vi "Sort Goal Info.vi"(0 "Distances Info":T2(array[cluster])) -> (1 "Left Goal":T3, 2 "Right Goal":T3)   [LabVIEW 2013]
uses:
  Common Code/Goal Info.ctl
  Vision/Goal Detection/TargetType.ctl
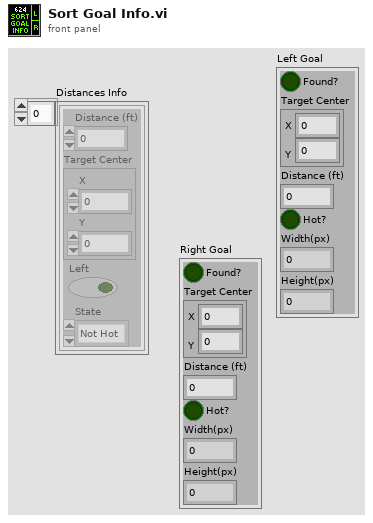
[diagram p1: front panel]
types:
  T1 = typedef "TargetType.ctl" = enum16{"Not Hot", "Hot"}
  T2 = cluster{"Distance (ft)":dbl, "Target Center":cluster{"X":dbl, "Y":dbl}, "Left":bool, "State":T1}[]
  T3 = typedef "Goal Info.ctl" = cluster{"Found?":bool, "Target Center":cluster{"X":dbl, "Y":dbl}, "Distance (ft)":dbl, "Hot?":bool, "Width(px)":dbl, "Height(px)":dbl}
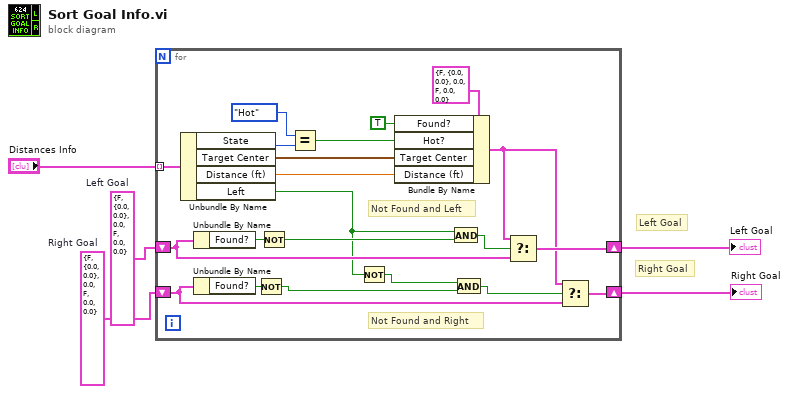
[diagram p0: block diagram]
diagram:
  w3 = T3 {"Found?"=FALSE, "Target Center"={"X"=0.0, "Y"=0.0}, "Distance (ft)"=0.0, "Hot?"=FALSE, "Width(px)"=0.0, "Height(px)"=0.0}  # Right Goal
  w2 = T3 {"Found?"=FALSE, "Target Center"={"X"=0.0, "Y"=0.0}, "Distance (ft)"=0.0, "Hot?"=FALSE, "Width(px)"=0.0, "Height(px)"=0.0}  # Left Goal
  # "Right Goal"
  # "Left Goal"
  n1 = for {
    tunnel: "Distances Info" -> [w26] mode=indexing
    shift-right: [w15] -> w4
    shift-left: w2 -> [w16]
    shift-right: [w18] -> w5
    shift-left: w3 -> [w17]
    # "Not Found and Right"
    # "Not Found and Left"
    n2 = Unbundle By Name(w26) -> ("State"=w25:T1, "Target Center"=w20:cluster{"X":dbl, "Y":dbl}, "Distance (ft)"=w19:dbl, "Left"=w10:bool)
    n3 = Unbundle By Name(w16) -> ("Found?"=w13:bool)
    n4 = Unbundle By Name(w17) -> ("Found?"=w12:bool)
    n5 = Not(x=w12) -> (.not. x?=w8:bool)
    n6 = Not(x=w13) -> (.not. x?=w11:bool)
    n7 = Equal?(x=TargetType."Hot", y=w25) -> (x = y?=w21:bool)
    n8 = Not(x=w10) -> (.not. x?=w9:bool)
    n9 = Bundle By Name(cluster=T3 {"Found?"=FALSE, "Target Center"={"X"=0.0, "Y"=0.0}, "Distance (ft)"=0.0, "Hot?"=FALSE, "Width(px)"=0.0, "Height(px)"=0.0}, "Found?"=TRUE, "Hot?"=w21, "Target Center"=w20, "Distance (ft)"=w19) -> (w7:T3)
    n10 = And(x=w10, y=w11) -> (x .and. y?=w14:bool)
    n11 = And(x=w9, y=w8) -> (x .and. y?=w6:bool)
    n12 = Select(t=w7, s=w14, f=w16) -> (s? t:f=w15:T3)
    n13 = Select(t=w7, s=w6, f=w17) -> (s? t:f=w18:T3)
  }
  "Right Goal" <- w5
  "Left Goal" <- w4
